vi "Host Keyboard.vi"() -> ()   [LabVIEW 2015]
uses:
  TypeDefs Host/Keyboard.ctl
panel:
  in  "Stop Button":bool
  in  "Keyboard 2":T1
  in  "Keyboard":T1
  in  "Scale":u8(slide)=1 scale=0.0..10.0
  in  "SawSin":bool
  in  "Accu?":bool
  out "Freq":u16
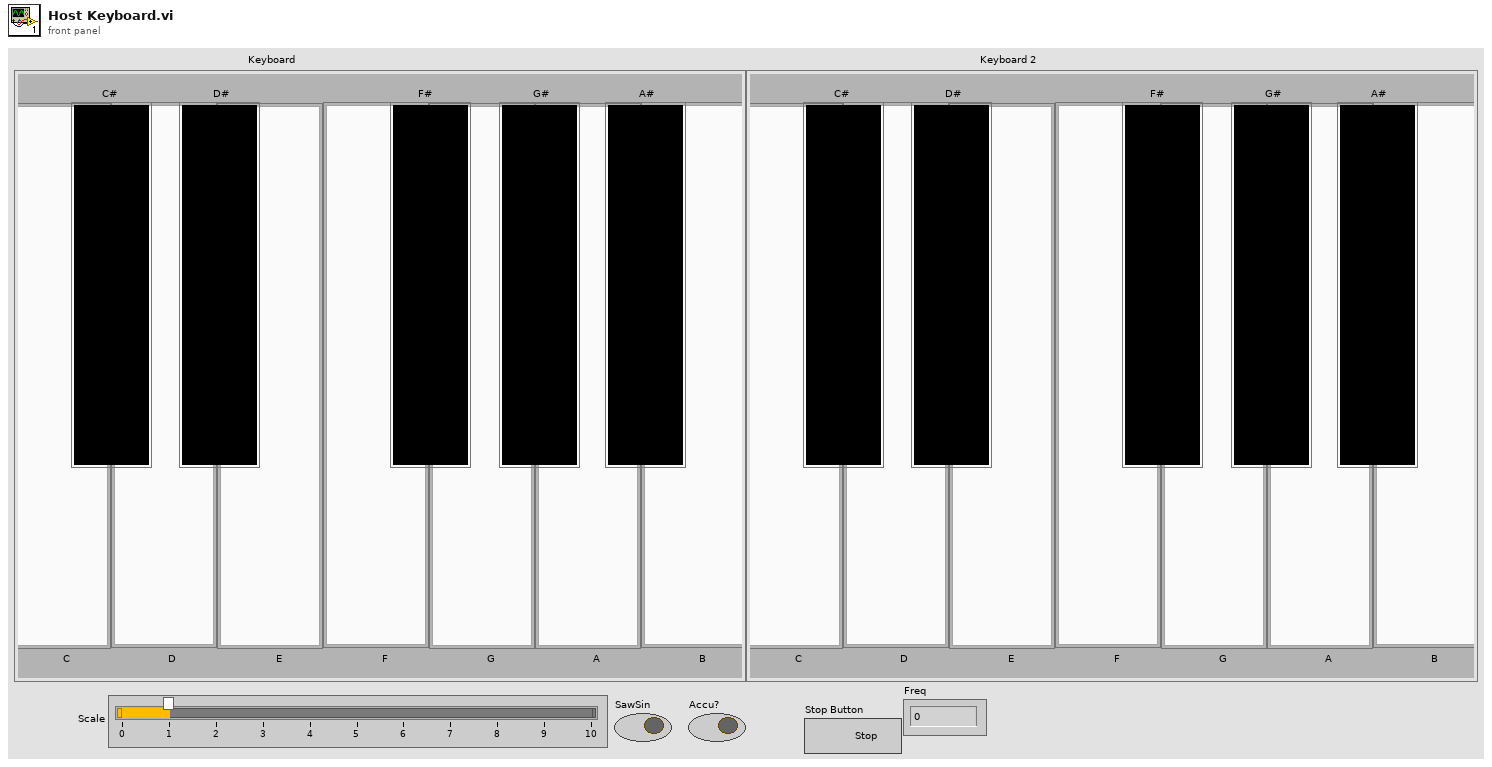
[diagram p1: front panel]
types:
  T1 = typedef "Keyboard.ctl" = cluster{"C":bool, "C#":bool, "D":bool, "D#":bool, "E":bool, "F":bool, "F#":bool, "G":bool, "G#":bool, "A":bool, "A#":bool, "B":bool}
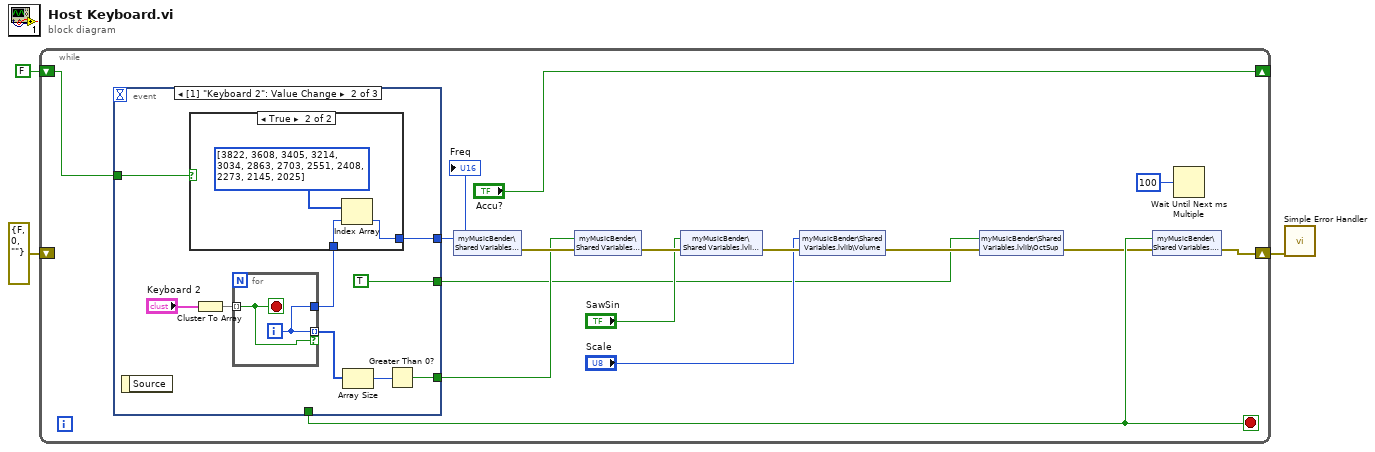
[diagram p0: block diagram]
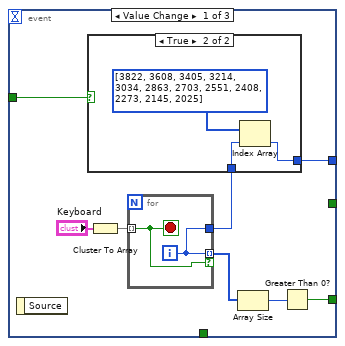
[diagram p2: hidden frame]
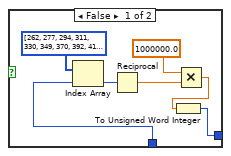
[diagram p3: hidden frame]
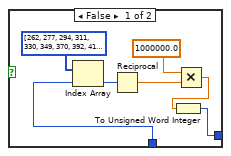
[diagram p4: hidden frame]
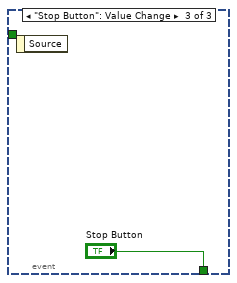
[diagram p5: hidden frame]
diagram:
  n1 = while {
    shift-right: [w14] -> w2
    shift-left: errorcluster {"status"=FALSE, "code"=0, "source"=""} ("error IO") -> [_]
    shift-right: ["Accu?"] -> _
    shift-left: FALSE ("Accu?") -> [w4]
    stop <- w11 stop-if-true
    n2 = event shown="[1] \"Keyboard 2\": Value Change" {
      selector: _ -> [_ _ _]
      dyn-events: _ -> [_ _ _]
      timeout: _ -> [_ _ _]
      tunnel: [w20 w43 _] -> w17
      tunnel: [w22 w42 _] -> w15
      tunnel: [_ _ "Stop Button"] -> w11
      tunnel: [_ TRUE ("Octava Sup") _] -> w6
      tunnel: w4 -> [w19 w39 _]
      event Value Change {
        n3 = event-data() -> ()  [unwired: 1 in, 1 out]
        n4 = Cluster To Array(cluster="Keyboard") -> (array=w26:bool[])
        n5 = for {
          tunnel: [w38] -> w21
          tunnel: w26 -> [w37] mode=indexing
          tunnel: [w38] -> w24 mode=indexing if=w37
          i -> [w38]
          stop <- w37 stop-if-true
        }
        n6 = case shown="True" w19 {
          tunnel: w21 -> [w33 w35]
          tunnel: [w28 w34] -> w20
          frame False {
            n7 = Index Array(array=u16[] [262, 277, 294, 311, 330, 349, 370, 392, 415, 440, 466, 494], index=w33) -> (element=w31:u16)
            n8 = Reciprocal(x=w31) -> (1/x=w30:dbl)
            n9 = Multiply(x=1000000.0, y=w30) -> (x*y=w27:dbl)
            n10 = To Unsigned Word Integer(number=w27) -> (unsigned 16bit integer=w28:u16)
          }
          frame True {
            n11 = Index Array(array=u16[] [3822, 3608, 3405, 3214, 3034, 2863, 2703, 2551, 2408, 2273, 2145, 2025], index=w35) -> (element=w34:u16)
          }
        }
        n12 = Array Size(array=w24) -> (size(s)=w23:i32)
        n13 = Greater Than 0?(x=w23) -> (x > 0?=w22:bool)
      }
      event Value Change {
        n14 = event-data() -> ()  [unwired: 1 in, 1 out]
        n15 = Cluster To Array(cluster="Keyboard 2") -> (array=w46:bool[])
        n16 = for {
          tunnel: [w59] -> w47
          tunnel: w46 -> [w58] mode=indexing
          tunnel: [w59] -> w45 mode=indexing if=w58
          i -> [w59]
          stop <- w58 stop-if-true
        }
        n17 = case shown="True" w39 {
          tunnel: w47 -> [w54 w56]
          tunnel: [w49 w55] -> w43
          frame False {
            n18 = Index Array(array=u16[] [262, 277, 294, 311, 330, 349, 370, 392, 415, 440, 466, 494], index=w54) -> (element=w52:u16)
            n19 = Reciprocal(x=w52) -> (1/x=w51:dbl)
            n20 = Multiply(x=1000000.0, y=w51) -> (x*y=w48:dbl)
            n21 = To Unsigned Word Integer(number=w48) -> (unsigned 16bit integer=w49:u16)
          }
          frame True {
            n22 = Index Array(array=u16[] [3822, 3608, 3405, 3214, 3034, 2863, 2703, 2551, 2408, 2273, 2145, 2025], index=w56) -> (element=w55:u16)
          }
        }
        n23 = Array Size(array=w45) -> (size(s)=w44:i32)
        n24 = Greater Than 0?(x=w44) -> (x > 0?=w42:bool)
      }
      event "Stop Button": Value Change {
        n25 = event-data() -> ()  [unwired: 1 in, 1 out]
      }
    }
    "Freq" <- w17
    n26 = shared-variable "myMusicBender\\Shared Variables.lvlib\\Freq"(w17) -> (error out=w16:errorcluster)  [unwired: 1 in]
    n27 = shared-variable "myMusicBender\\Shared Variables.lvlib\\Play"(w15, error in=w16) -> (error out=w13:errorcluster)
    n28 = shared-variable "myMusicBender\\Shared Variables.lvlib\\SawSin"("SawSin", error in=w13) -> (error out=w12:errorcluster)
    n29 = shared-variable "myMusicBender\\Shared Variables.lvlib\\Volume"("Scale", error in=w12) -> (error out=w10:errorcluster)
    n30 = shared-variable "myMusicBender\\Shared Variables.lvlib\\OctSup"(w6, error in=w10) -> (error out=w9:errorcluster)
    n31 = shared-variable "myMusicBender\\Shared Variables.lvlib\\Stop"(w11, error in=w9) -> (error out=w14:errorcluster)
    n32 = Wait Until Next ms Multiple(millisecond multiple=u32 100) -> ()  [unwired: 1 out]
  }
  n33 = call <vilib>:"Simple Error Handler.vi"("error in (no error)"=w2) -> ()  [unwired: 4 in, 5 out]
